vi "Get Result.vi"(8 "error in (no error)":errorcluster, 11 "Mag Lab Root in":refnum<class "Mag Lab Root.lvclass">) -> (0 "error out":errorcluster, 2 "Result":refnum<class "Mag Lab Result.lvclass">, 3 "Mag Lab Root out":refnum<class "Mag Lab Root.lvclass">)   [LabVIEW 2015, in "Mag Lab Root.lvclass"]
uses:
  Mag Lab Root.lvclass
  Mag Lab Result/Mag Lab Result.lvclass
  Mag Lab Root.lvclass/Mag Lab Root.ctl
  Mag Lab Result/Mag Lab Result.lvclass/Mag Lab Result.ctl
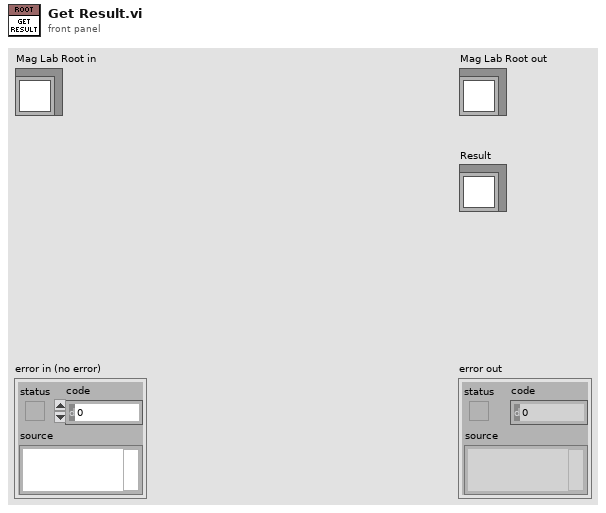
[diagram p1: front panel]
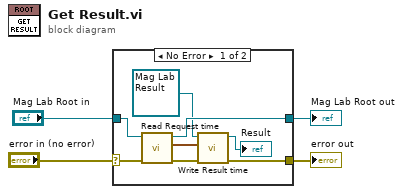
[diagram p0: block diagram]
diagram:
  n1 = case shown="No Error" "error in (no error)" {
    selector: "error in (no error)" -> [w8 w14]
    tunnel: [w6 w14] -> w3
    tunnel: [w11 w13] -> w1
    tunnel: "Mag Lab Root in" -> [w12 w13]
    frame No Error {
      n2 = call "Read Request time.vi"("error in (no error)"=w8, "Mag Lab Root in"=w12) -> ("error out"=w7:errorcluster, "Request time"=w9:timestamp, "Mag Lab Root out"=w11:refnum<class "Mag Lab Root.lvclass">)  [unwired: 7 in]
      n3 = call "Write Result time.vi"("error in (no error)"=w7, "Result time"=w9, "Mag Lab Result in"=refnum<class "Mag Lab Result.lvclass"> refnum ("Result")) -> ("error out"=w6:errorcluster, "Mag Lab Result out"=→"Result":refnum<class "Mag Lab Result.lvclass">)  [unwired: 7 in]
    }
    frame Error {
    }
  }
  "error out" <- w3
  "Mag Lab Root out" <- w1
